vi "_convert_response_to_integer_scalar_number.vi"(8 "error in":errorcluster caption="error in (no error)", 10 "Input string":string, 11 "VISA resource name":refnum<visa-resource-name>) -> (0 "error out":errorcluster, 2 "Int32 out":i32, 3 "VISA resource name out":refnum<visa-resource-name>)   [LabVIEW 2020, in "Rohde&Schwarz RTx Oscilloscopes.lvlib" / "rsidr_core.lvlib"]
doc: "Queries array of floats that can be returned in ASCII format or in binary format. The array is always returned as the most-universal double array.\n- For <b>ASCII</b> format, the array numbers are decoded as comma-separated values.\n- For <b>Binary Format</b>, the numbers are decoded based on the session parameter <b>Bin Float Number Format</b>, usually float 32-bit (REAL,32), swapped endianess (instruments usually use low endian, LabVIEW uses big endian)."
uses:
  rsidr_core.lvlib
  type_AdditionalFlag_Bits.ctl
  type_Error_Codes.ctl
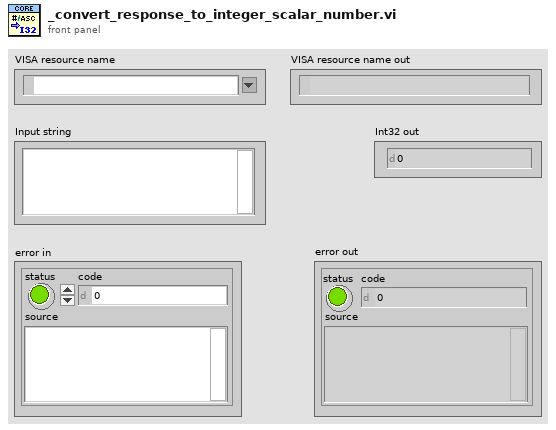
[diagram p1: front panel]
types:
  T1 = typedef "Rohde&Schwarz RTx Oscilloscopes.lvlib/rsidr_core.lvlib/type_AdditionalFlag_Bits.ctl" = enum16{"Send LF after Bin Block", "Junk read with io_clear_buffers.vi", "io_clear_buffers: viClear()", "io_clear_buffers: viFlush()", "<NotUsed1>", "Allow Dbl & Int Bin/Ascii read", "*OPC? in check_instrument_error.vi", "<NotUsed2>", "Smart Enum Matching", "Less Strict RepCaps check", "AssureResponseEndWithLF"}
  T2 = typedef "Rohde&Schwarz RTx Oscilloscopes.lvlib/rsidr_core.lvlib/type_Error_Codes.ctl" = enum16{"No_error", "VISA_err_ResourceNotFound", "VISA_err_Timeout", "VISA_warn_MoreDataAvailable", "RS_err_MissingCallback", "RS_err_InvalidAttribute", "RS_err_InvalidValue", "RS_err_UnknownResource", "RS_err_AlreadyInitialized", "RS_err_InstrumentStatus", "RS_err_BadRepCapName", "RS_err_TypesMismatch", "RS_err_ValueNotSupported", "RS_err_InvalidRngTable", "RS_err_IDqueryFail", "RS_err_UnexpResponse", "VISA_warn_ConfigNotLoaded", "RS_err_AttributeNotReadable", "RS_err_AttributeNotWritable", "RS_err_InstrumentType", "RS_err_InstrumentOption", "VISA_err_InvalidSize", "RS_err_ReliabilityIndicator", "VISA_warn_UnknownStatus", "VISA_warn_TermCharRead", "VISA_err_IO_error", "RS_err_FunctionNotSupported", "VISA_warn_QueueEmpty"}
  T3 = typedef "Rohde&Schwarz RTx Oscilloscopes.lvlib/rsidr_core.lvlib/type_Session_Data.ctl" = cluster{"IDN string":string, "Instrument FW":string, "Instr type":string, "Instr type for err. msg.":string, "Installed Options":string[], "Ignore Error Messages":string, "Logging params":variant, "OPC Timeout":i32, "VISA Timeout":i32, "STB Poll VISA Timeout":i32, "Additional Flags":i32, "Wait Before Read":i32, "Wait Before Write":i32, "Option String Flags":i32, "IO Segment Size":i64, "VISA Access Mode":T4, "Interface Type":T5, "OPC Wait Mode":T6, "Bin Float Number  Format":T7, "Bin Integer Number Format":T8, "Simulate":bool, "VXIcapable":bool, "Duplicate Session":bool, "Add LF to Write":bool, "Logging":bool, "Fast Sweep":bool, "Query Instrument Status":bool, "Check Range":bool, "Check Options":bool, "OPC-sync Attr Writes":bool, "OPC-sync Attr Queries":bool}
  T4 = typedef "Rohde&Schwarz RTx Oscilloscopes.lvlib/rsidr_core.lvlib/type_VisaAccessMode.ctl" = u16
  T5 = typedef "Rohde&Schwarz RTx Oscilloscopes.lvlib/rsidr_core.lvlib/type_InterfaceType.ctl" = enum16{"Unknown", "GPIB", "VXI", "GPIB_VXI", "ASRL", "PXI", "TCPIP", "USB", "SOCKET"}
  T6 = typedef "Rohde&Schwarz RTx Oscilloscopes.lvlib/rsidr_core.lvlib/type_OPC_Wait_Mode.ctl" = enum16{"STBpolling", "STBpollingSlow", "STBpollingSuperSlow", "ServiceRequest", "OPCquery"}
  T7 = typedef "Rohde&Schwarz RTx Oscilloscopes.lvlib/rsidr_core.lvlib/type_Binary_Float_Number_Format.ctl" = enum16{"Float_4_Bytes_Swapped", "Float_4_Bytes", "Double_8_Bytes_Swapped", "Double_8_Bytes"}
  T8 = typedef "Rohde&Schwarz RTx Oscilloscopes.lvlib/rsidr_core.lvlib/type_Binary_Integer_Number_Format.ctl" = enum16{"Int32_4_Bytes_Swapped", "Int32_4 Bytes", "Int16_2_Bytes_Swapped", "Int16_2_Bytes"}
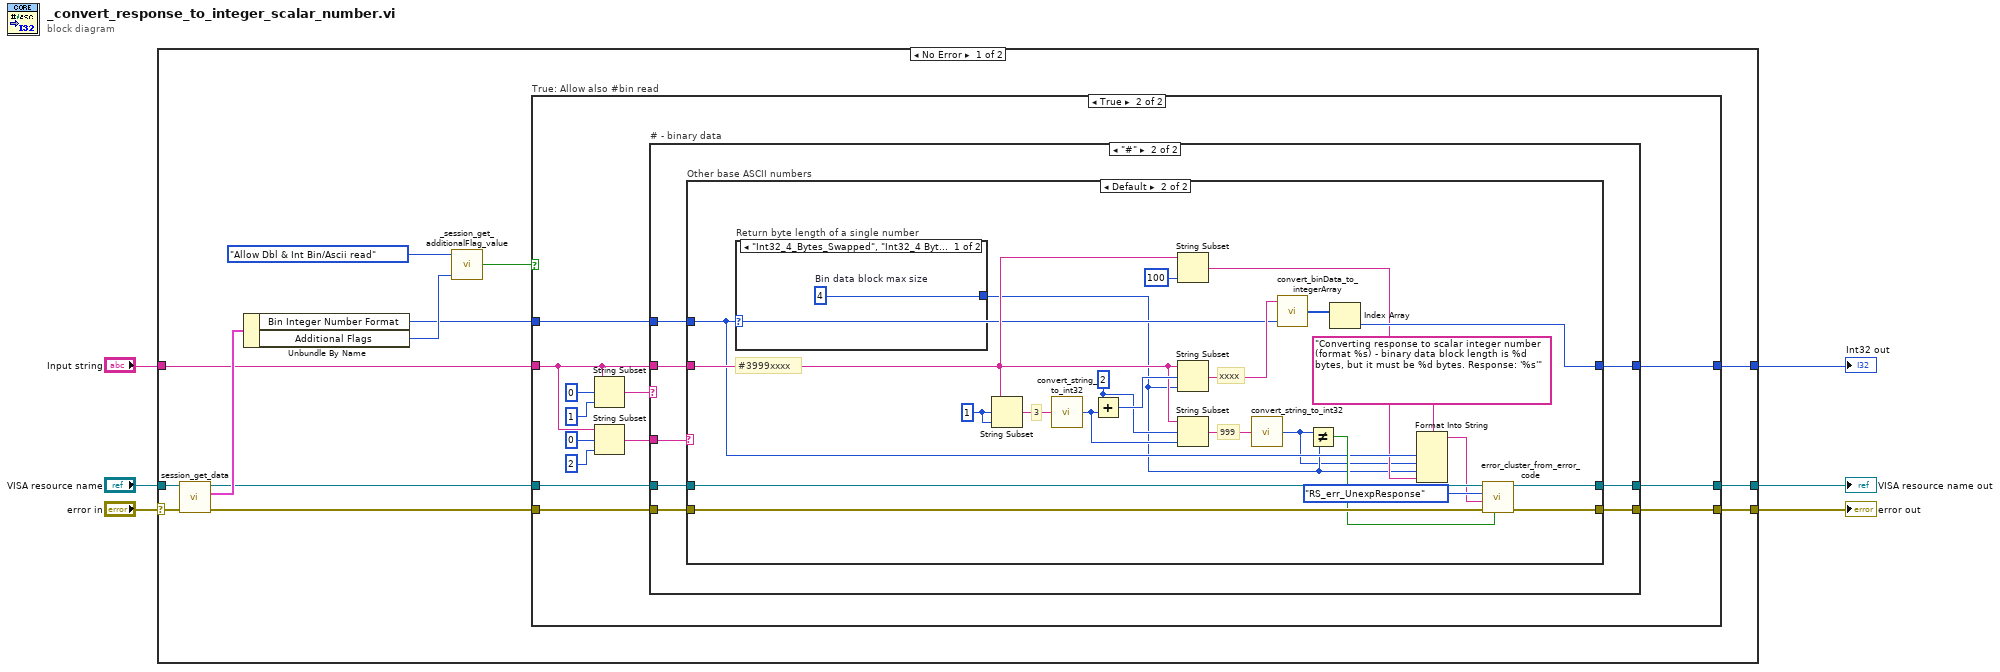
[diagram p0: block diagram]
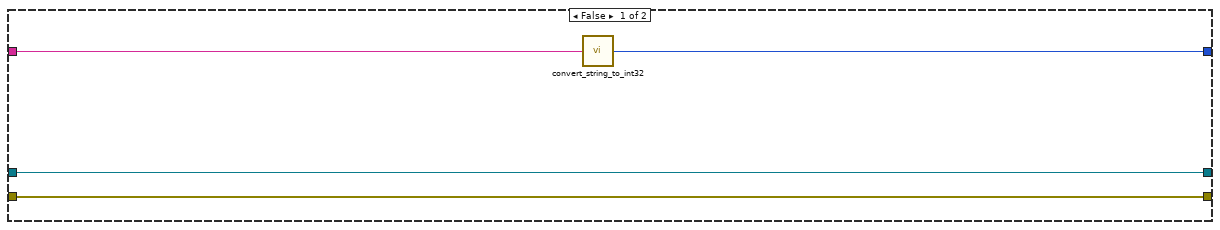
[diagram p2: hidden frame]
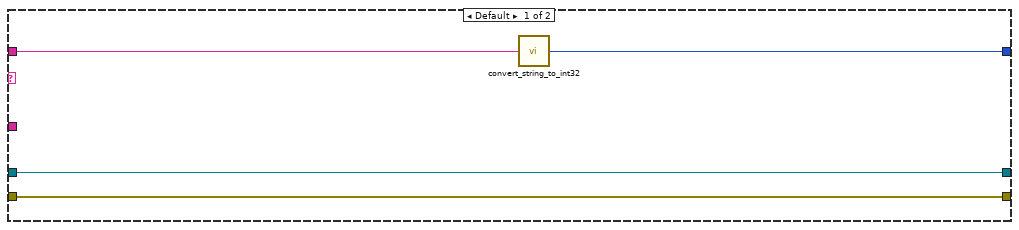
[diagram p3: hidden frame]
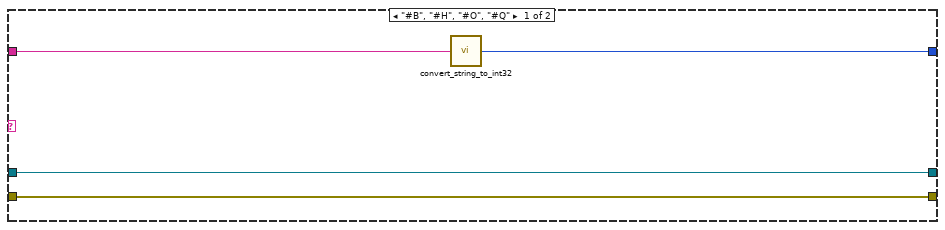
[diagram p4: hidden frame]
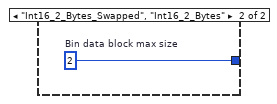
[diagram p5: hidden frame]
diagram:
  n1 = case shown="No Error" "error in" {
    selector: "error in" -> [w19 w79]
    tunnel: [w8 w78] -> w1
    tunnel: [w9 w79] -> w2
    tunnel: "VISA resource name" -> [w18 w78]
    tunnel: [w13 _] -> w3
    tunnel: "Input string" -> [w12 _]
    frame No Error {
      n2 = call "session_get_data.vi"("error in"=w19, "VISA resource name"=w18) -> ("error out"=w11:errorcluster, "Session User Data out"=w17:T3, "VISA resource name out"=w10:refnum<visa-resource-name>)  [unwired: 6 in, 1 out]
      n3 = Unbundle By Name(w17) -> ("Bin Integer Number Format"=w7:T8, "Additional Flags"=w15:i32)
      n4 = call "_session_get_additionalFlag_value.vi"("AdditionalFlags value in"=w15, "AdditionalFlag bit"=type_AdditionalFlag_Bits."Allow Dbl & Int Bin/Ascii read") -> ("AdditionalFlag bit value out"=w14:bool)  [unwired: 3 in]
      n5 = case "True: Allow also #bin read" shown="True" w14 {
        tunnel: w7 -> [_ w29]
        tunnel: [w22 w34] -> w13
        tunnel: w12 -> [w23 w26]
        tunnel: w11 -> [w21 w33]
        tunnel: w10 -> [w20 w32]
        tunnel: [w21 w31] -> w9
        tunnel: [w20 w30] -> w8
        frame False {
          n6 = call "convert_string_to_int32.vi"("String in"=w23) -> ("int32 value out"=w22:i32)  [unwired: 4 in]
        }
        frame True {
          n7 = String Subset(string=w26, offset (0)=0, length (rest)=1 ("length (rest)")) -> (substring=w25:string)
          n8 = String Subset(string=w26, offset (0)=0, length (rest)=2 ("length (rest)")) -> (substring=w24:string)
          n9 = case "# - binary data" shown="\"#\"" w25 {
            tunnel: w26 -> [w40 w43]
            tunnel: w29 -> [_ w42]
            tunnel: [w39 w48] -> w34
            tunnel: w33 -> [w38 w47]
            tunnel: w32 -> [w37 w46]
            tunnel: [w38 w45] -> w31
            tunnel: [w37 w44] -> w30
            tunnel: w24 -> [_ w41]
            frame Default {
              n10 = call "convert_string_to_int32.vi"("String in"=w40) -> ("int32 value out"=w39:i32)  [unwired: 4 in]
            }
            frame "#" {
              n11 = case "Other base ASCII numbers" shown="Default" w41 {
                tunnel: [w51 w71] -> w48
                tunnel: w47 -> [w50 w65]
                tunnel: w46 -> [w49 w64]
                tunnel: [w50 w63] -> w45
                tunnel: [w49 w62] -> w44
                tunnel: w43 -> [w52 w58]
                tunnel: w42 -> [_ w56]
                frame "#B", "#H", "#O", "#Q" {
                  n12 = call "convert_string_to_int32.vi"("String in"=w52) -> ("int32 value out"=w51:i32)  [unwired: 4 in]
                }
                frame Default {
                  w69 = 2 ("offset (0)")
                  w75 = 1 ("offset (0)")
                  # "xxxx"
                  # "999"
                  # "3"
                  # "#3999xxxx"
                  n13 = case "Return byte length of a single number" shown="\"Int32_4_Bytes_Swapped\", \"Int32_4 Bytes\"" w56 {
                    tunnel: [w76 w77] -> w54
                    frame "Int32_4_Bytes_Swapped", "Int32_4 Bytes" {
                      w76 = 4  # Bin data block max size
                    }
                    frame "Int16_2_Bytes_Swapped", "Int16_2_Bytes" {
                      w77 = 2  # Bin data block max size
                    }
                  }
                  n14 = String Subset(string=w58, offset (0)=w75, length (rest)=w75) -> (substring=w74:string)
                  n15 = call "convert_string_to_int32.vi"("String in"=w74) -> ("int32 value out"=w68:i32)  [unwired: 4 in]
                  n16 = Add(x=w69, y=w68) -> (x+y=w70:i32)
                  n17 = String Subset(string=w58, length (rest)=100 ("length (rest)")) -> (substring=w55:string)  [unwired: 1 in]
                  n18 = String Subset(string=w58, offset (0)=w70, length (rest)=w54) -> (substring=w73:string)
                  n19 = String Subset(string=w58, offset (0)=w69, length (rest)=w68) -> (substring=w67:string)
                  n20 = call "convert_string_to_int32.vi"("String in"=w67) -> ("int32 value out"=w53:i32)  [unwired: 4 in]
                  n21 = call "convert_binData_to_integerArray.vi"("Bin Number Integer Format"=w56, "Bin Data"=w73) -> ("Numbers out"=w72:i32[])  [unwired: 1 in, 2 out]
                  n22 = Not Equal?(x=w53, y=w54) -> (x != y?=w61:bool)
                  n23 = Index Array(array=w72) -> (element=w71:i32)  [unwired: 1 in]
                  n24 = Format Into String(format string="Converting response to scalar integer number (format %s) - binary data block length is %d bytes, but it must be %d bytes. Response: '%s'", w56, w53, w54, w55) -> (resulting string=w59:string)  [unwired: 2 in, 1 out]
                  n25 = call "error_cluster_from_error_code.vi"("Error Creation Enabled (True)"=w61, "error in"=w65, "Error Message (\"\")"=w59, "Error Enum in"=type_Error_Codes."RS_err_UnexpResponse", "VISA resource name"=w64) -> ("error out"=w63:errorcluster, "VISA resource name out"=w62:refnum<visa-resource-name>)  [unwired: 5 in]
                }
              }
            }
          }
        }
      }
    }
    frame Error {
    }
  }
  "error out" <- w2
  "VISA resource name out" <- w1
  "Int32 out" <- w3
